vi "niScope Initialize.vi"(0 "resource name":refnum<k15>, 5 "id query":bool, 9 "reset device":bool=TRUE, 11 "error in":errorcluster) -> (4 "instrument handle":refnum<k15>, 15 "error out":errorcluster)   [LabVIEW 2020]
doc: "Performs the following initialization actions:\n\n-Creates a new IVI instrument driver session.\n\n-Opens a session to the device(s) that you specify in the resource name parameter.\n\n-Queries each instrument ID and verifies that it is valid for this instrument driver.\n\n-Resets the instrument(s) to a known state if the reset device parameter is set to TRUE; refer to niScope Reset for the default state of each digitizer.\n\n-Sends initialization commands to set the instrument(s) to the state necessary for the operation of the instrument driver.\n\n-Returns an instrument handle that you use to identify the instrument(s) in all subsequent instrument driver VI calls."
uses:
  niScope_32.dll
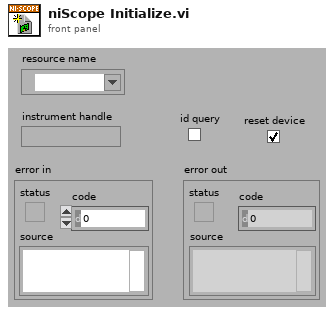
[diagram p1: front panel]
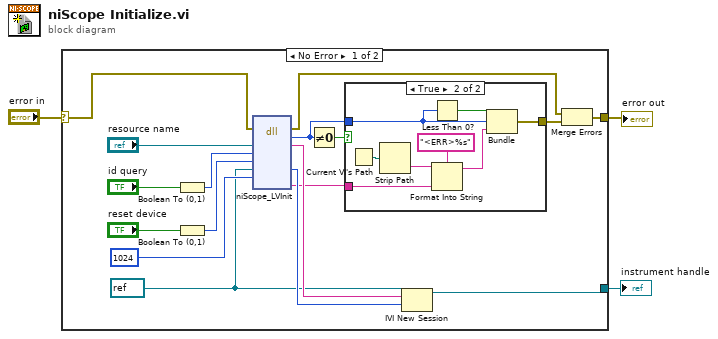
[diagram p0: block diagram]
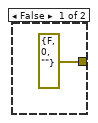
[diagram p2: hidden frame]
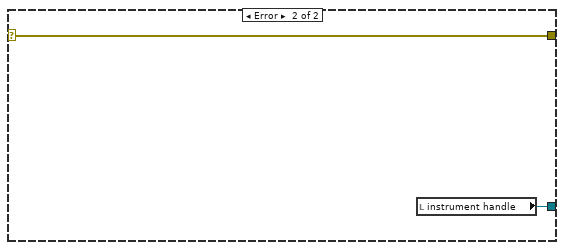
[diagram p3: hidden frame]
diagram:
  n1 = case shown="No Error" "error in" {
    selector: "error in" -> [w5 w30]
    tunnel: [w7 w30] -> w3
    tunnel: [w15 w31] -> w2
    frame No Error {
      w6 = refnum<k15> refnum
      n2 = Boolean To (0,1)(Boolean="id query") -> (0, 1=w17:i16)
      n3 = Boolean To (0,1)(Boolean="reset device") -> (0, 1=w16:i16)
      n4 = dll-call lib="niScope_*.*" fn="niScope_LVInit"(error in=w5, "resourceName"="resource name", "IDQuery"=w17, "resetDevice"=w16, "instrument handle"=w6, "error buffer size"=1024) -> (error out=w4:errorcluster, "status"=w11:i32, "resourceName"=w14:string, "instrument handle"=w13:u32, "error buffer"=w9:string)  [unwired: 6 in, 1 out]
      n5 = Not Equal To 0?(x=w11) -> (x != 0?=w12:bool)
      n6 = case shown="True" w12 {
        tunnel: w9 -> [_ w29]
        tunnel: w11 -> [_ w24]
        tunnel: [cluster{bool, "status":i32, string} {FALSE, "status"=0, ""} w22] -> w8
        frame False {
        }
        frame True {
          n7 = Current VI's Path() -> (path=w27:path)
          n8 = Strip Path(path=w27) -> (name=w26:string)  [unwired: 1 out]
          n9 = Less Than 0?(x=w24) -> (x < 0?=w23:bool)
          n10 = Format Into String(format string="<ERR>%s", initial string=w26, w29) -> (resulting string=w25:string)  [unwired: 1 in, 1 out]
          n11 = Bundle(w23, "status"=w24, w25) -> (w22:cluster{bool, "status":i32, string})  [unwired: 1 in]
        }
      }
      n12 = IVI New Session(9:w13, 10:w14, 11:w6) -> (3:w15:refnum<k15>)
      n13 = Merge Errors(w4, w8) -> (w7:errorcluster)
    }
    frame Error {
      n14 = local read "instrument handle"() -> (w31:refnum<k15>)
    }
  }
  "error out" <- w3
  "instrument handle" <- w2
